vi "MyRIO Lidar Read Data.vi"(8 "error in (no error)":errorcluster={"status"=FALSE, "code"=2, "source"="Lidar Failed to init"}) -> (0 "error out":errorcluster={"status"=FALSE, "code"=2, "source"="Lidar Failed to init"}, 2 "Lidar Data":T1={"Directions (rads)"=array[484 elements], "Magnitudes"=[832, 832, 832, 825, 819, 808, 807, 807, 808, 804, 807, 807, 807, 806, 793, 790, 786, 783, 783, 781, 781, 777, 775, 777, 777, 777, 772, 772, 771, 772, 771, 771, 772, 780, 770, 770, 770, 770, 770, 770, 770, 757, 754, 757, 757, 758, 759, 760, 765, 759, 766, 771, 766, 757, 766, 768, 768, 769, 769, 769, 769, 766, 766, 766, 766, 766, 773, 773, 773, 773, 770, 767, 765, 765, 767, 768, 768, 767, 767, 767, 768, 770, 770, 770, 761, 761, 761, 763, 764, 764, 763, 767, 767, 767, 767, 767, 780, 768, 764, 770, 770, 764, 764, 772, 763, 765, 765, 765, 765, 774, 779, 779, 779, 779, 779, 779, 780, 784, 784, 788, 790, 788, 790, 790, 788, 788, 791, 791, 792, 793, 799, 803, 803, 803, 803, 804, 804, 809, 809, 812, 812, 812, 813, 813, 822, 822, 822, 827, 831, 831, 831, 838, 838, 839, 851, 851, 854, 855, 861, 844, 866, 872, 877, 882, 882, 882, 882, 884, 885, 897, 897, 898, 899, 899, 904, 911, 912, 912, 916, 933, 933, 937, 938, 944, 949, 962, 963, 964, 965, 969, 972, 975, 985, 988, 1000, 1006, 1006, 1014, 1017, 1027, 1031, 1035, 1048, 1049, 1066, 1067, 1069, 1076, 1087, 1093, 1099, 1113, 1118, 1132, 1135, 1144, 1153, 1167, 1174, 1177, 1184, 1197, 1232, 1226, 1239, 1263, 1275, 1288, 1307, 1313, 1316, 1334, 1344, 1348, 1364, 1370, 1381, 1381, 1381, 1377, 1370, 1364, 1362, 1354, 1354, 1341, 1339, 1331, 1329, 1327, 1322, 1320, 1313, 1310, 1300, 1297, 1295, 1292, 1291, 1286, 1285, 1282, 1279, 1279, 1275, 1265, 1265, 1260, 1257, 1256, 1250, 1246, 1244, 1244, 1244, 1244, 1244, 1239, 1236, 1236, 1235, 1233, 1227, 1227, 1222, 1235, 1217, 1216, 1214, 1207, 1204, 1204, 1204, 1204, 1201, 1201, 1201, 1200, 1199, 1199, 1199, 1198, 1198, 1198, 1198, 1192, 1192, 1190, 1192, 1192, 1188, 1198, 1198, 1198, 1197, 1197, 1194, 1193, 1193, 1194, 1194, 1194, 1197, 1197, 1196, 1194, 1190, 1190, 1189, 1189, 1189, 1190, 1191, 1191, 1199, 1199, 1199, 1196, 1196, 1194, 1194, 1194, 1192, 1194, 1194, 1195, 1199, 1199, 1170, 1195, 1196, 1193, 1196, 1196, 1201, 1203, 1203, 1203, 1203, 1201, 1201, 1201, 1203, 1206, 1208, 1208, 1214, 1215, 1219, 1219, 1219, 1220, 1223, 1223, 1229, 1230, 1230, 1232, 1232, 1237, 1242, 1244, 1251, 1254, 1255, 1257, 1262, 1265, 1268, 1273, 1274, 1281, 1283, 1293, 1296, 1298, 1298, 1305, 1310, 1313, 1319, 1320, 1325, 1325, 1329, 1338, 1339, 1345, 1356, 1357, 1359, 1363, 1373, 1377, 1379, 1390, 1397, 1404, 1411, 1412, 1429, 1433, 1434, 1447, 1458, 1458, 1468, 1474, 1479, 1485, 1485, 1512, 1513, 1515, 1522, 1528, 1538, 1539, 1557, 1577, 1579, 1582, 1603, 1606, 1610, 1629, 1648, 1658, 1667, 1669, 1683, 1705, 1708, 1709, 1743, 1743, 1743, 1737, 1728, 1727, 1678, 1672, 1663, 1643, 1637, 1629, 1628, 1623, 1597, 1593, 1587, 1587, 1582, 1561, 1562, 1554, 1550, 1549, 1547, 1539, 1519, 1512, 1506, 1506]})   [LabVIEW 2016]
uses:
  Variables/MyRIO Lidar Class Data.vi
panel:
  in  "Angular resolution (rads)":dbl=0.006135923151542565
  in  "length":i32=492
  in  "index":i32=72
  in  "Angle offset":dbl=1.732
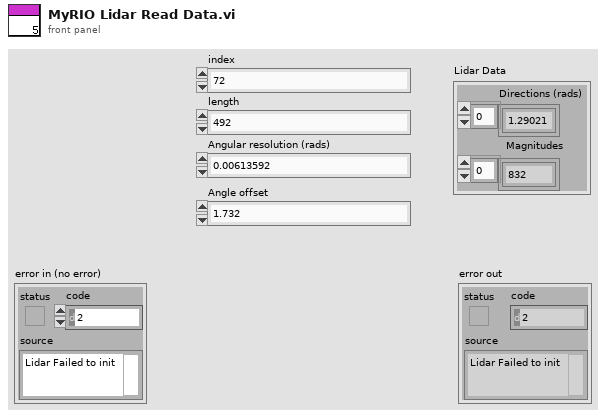
[diagram p1: front panel]
types:
  T1 = cluster{"Directions (rads)":dbl[], "Magnitudes":u16[]}
  T2 = cluster{"Shared library path":path, "File Descriptor":i32}
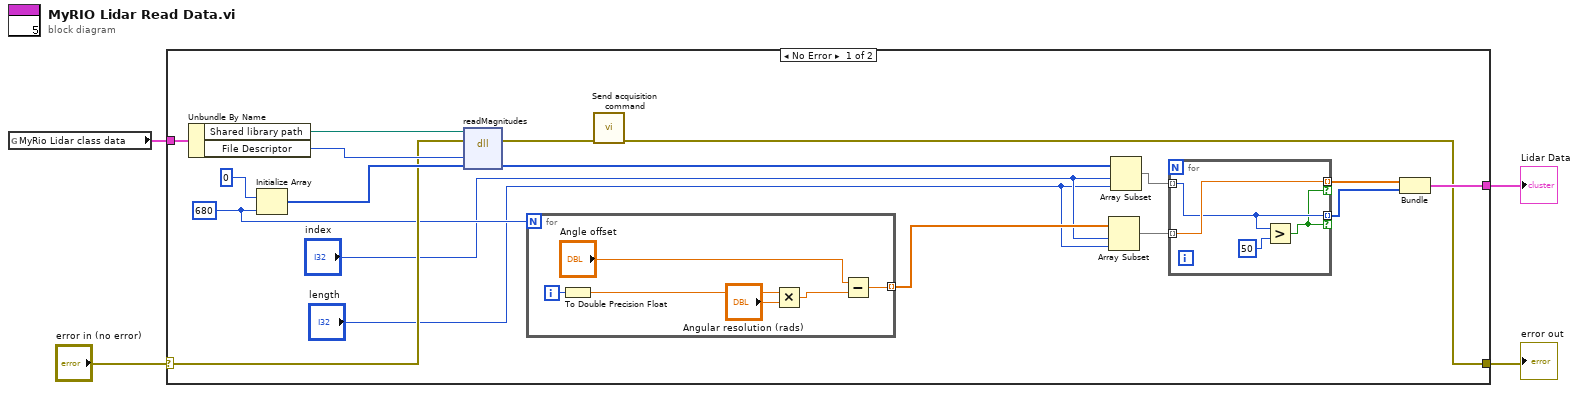
[diagram p0: block diagram]
diagram:
  n1 = global read "MyRIO Lidar Class Data.vi" "MyRio Lidar class data"() -> (w1:T2)
  n2 = case shown="No Error" "error in (no error)" {
    selector: "error in (no error)" -> [w16 w33]
    tunnel: [w13 w33] -> w3
    tunnel: w1 -> [w15 _]
    tunnel: [w17 _] -> w2
    frame No Error {
      w12 = 680 ("dimension size")
      n3 = Unbundle By Name(w15) -> ("Shared library path"=w19:path, "File Descriptor"=w18:i32)
      n4 = Initialize Array(0 ("element"), w12) -> (w22:i32[])
      n5 = dll-call lib="?" fn="readMagnitudes"(path in=w19, error in=w16, "fd"=w18, "magnitudes"=w22) -> (error out=w14:errorcluster, "magnitudes"=w20:i32[])  [unwired: 3 in, 1 out]
      n6 = for {
        N: w12 -> [_]
        tunnel: [w31] -> w11 mode=indexing
        i -> [w32]
        n7 = To Double Precision Float(number=w32) -> (double precision float=w28:dbl)
        n8 = Multiply(x=w28, y="Angular resolution (rads)") -> (x*y=w29:dbl)
        n9 = Subtract(x="Angle offset", y=w29) -> (x-y=w31:dbl)
      }
      n10 = call "Send acquisition command.vi"("error in (no error)"=w14) -> ("error out"=w13:errorcluster)  [unwired: 10 in]
      n11 = Array Subset(array=w11, index="index", length="length") -> (w6:dbl[])
      n12 = Array Subset(array=w20, index="index", length="length") -> (w7:i32[])
      n13 = for {
        tunnel: [w26] -> w8 mode=indexing if=w23
        tunnel: w7 -> [w25] mode=indexing
        tunnel: w6 -> [w26] mode=indexing
        tunnel: [w25] -> w5 mode=indexing if=w23
        n14 = Greater?(x=w25, y=50) -> (0:w23:bool)
      }
      n15 = Bundle(w8, w5) -> (w17:cluster{dbl[], i32[]})  [unwired: 1 in]
    }
    frame Error {
    }
  }
  "error out" <- w3
  "Lidar Data" <- w2
